vi "ABB global.vi"() -> ()   [LabVIEW 2017]
panel:
  in  "Temp report folder":path=path "C:/Program Files/National Instruments/LabVIEW 7.1/LabView 7.1 Apps/ABB motor test/report templates"
  in  "Camera Addresses":T1
  out "Video Display Folder":path
  in  "ChangeVIdStreamPath":path=path "C:/Program Files/National Instruments/LabVIEW 7.1/LabView 7.1 Apps/ABB motor test/report templates"
  in  "Temperature sensors":string[](array[string])
  in  "Efficiency Units":u16(ring) items=["METRIC", "IMPERIAL", "", "", ""]
  in  "Running Average levels (dB)":cluster{"Total":dbl, "Log":dbl}
  in  "Background Average levels (dB)":cluster{"Total":dbl, "Log":dbl}
  in  "Running Noise analysis":dbl[][](array[numeric])
  in  "Background Noise analysis":dbl[][](array[numeric])
  in  "Efficiency Standard":u16(ring) items=["IEC", "NEMA"]
  in  "Additional Mech Loss":dbl
  in  "Slip ring temperatures":cluster{"K":dbl, "L":dbl, "M ":dbl}[](array[cluster])
  in  "Specified Noise":dbl
  in  "Nose Limit":dbl
  in  "Effy Load Selection":bool[](array[boolean])
  in  "PF Remarks":string
  in  "Noise mtr type":i32
  in  "# noise points":i32
  in  "Heat run VT&CT":T2={"VT Primary"=0.0, "VT Secondary"=0.0, "CT  Primary"=0.0, "CT Secondary"=0.0, "Current Shunt"=enum."Internal", "Avg interval"=0.3}
  in  "Locked rotor VT&CT":T2={"VT Primary"=0.0, "VT Secondary"=0.0, "CT  Primary"=0.0, "CT Secondary"=0.0, "Current Shunt"=enum."Internal", "Avg interval"=0.3}
  in  "Noload VT&CT":T2={"VT Primary"=0.0, "VT Secondary"=0.0, "CT  Primary"=0.0, "CT Secondary"=0.0, "Current Shunt"=enum."Internal", "Avg interval"=0.3}
  in  "Webdaq Report":cluster{"Report":string, "Interval":string}={"Report"="Test_1", "Interval"="LastScan"}
  in  "Cool curve rdgs":T3(array[cluster])
  in  "report IDs":cluster{"Document #":string, "Revision":string}={"Document #"="1234H2345", "Revision"="1.1"}
  in  "VT and CT Ratios":T4={"VT Primary"=0.0, "VT Secondary"=0.0, "CT  Primary"=0.0, "CT Secondary"=0.0, "Current Shunt"=enum."Internal", "Averaging interval"=0.3}
  in  "Rotor Insulation Resistance":T5
  in  "Stator Insulation Resistance":T5
  in  "Heat run Type":enum16{"Full Load", "Partial- & No-Load"}(ring)
  in  "Altitude":dbl=1550.0
  in  "Max Wdg temp rise":dbl=85.0
  in  "No load run config":T6
  in  "Noise Levels":cluster{"Noise Before":dbl, "Noise During":dbl}
  in  "Pass Fail Entries":string[][](array[string])
  in  "Effiy entries":string[][](array[string])
  in  "Effy Configuration":T7 {"Loads (%Rated)" format="%#.0f"}
  in  "Temperature Scaling":dbl[][](array[numeric])
  in  "Bearing run config":T6
  in  "Instruments":string[][](array[string])
  in  "Heat run config":T6
  in  "Heat Run Results":cluster{"results":dbl[][], "Comments":string}[](array[cluster])
  in  "Personel":string[](array[string])
  in  "Tested by":string[](array[string])
  in  "Bearing Insp results":string[](array[string])
  in  "Bearing Image files":string[][](array[string])
  in  "Noise Image files":string[][](array[string])
  in  "Viewing test":bool
  in  "Current test":path
  in  "Report template":string
  in  "Noise results":dbl[][](array[numeric])
  in  "Bearing run results":dbl[][](array[numeric])
  in  "report template folder":path=path "C:/Program Files/National Instruments/LabVIEW 7.1/LabView 7.1 Apps/ABB motor test/report templates"
  in  "miscellaneous":string[](array[string])
  in  "Bearing Run Autordg":T8={"Thermal Stability (%)"=2.0, "Reading interval (mins)"=2.0}
  in  "Locked rotor temp. alloc":i32[](array[numeric])
  in  "NoLoad temp. alloc":i32[](array[numeric])
  in  "Temperature names":string[](array[string])
  in  "Temperature alloc":string[](array[string])
  in  "Heat Run Autordg":T9={"Thermal Stability (deg/hr)"=2.0, "Reading interval (mins)"=2.0}
  in  "Locked rotor test results":dbl[][](array[numeric])
  in  "Locked Rotor Autordg":T10={"Number Values"=8, "Tolerance"=2.0, "Value (ratio) "=[1.15, 1.0, 0.91, 0.78, 0.66, 0.55, 0.42, 0.3], "Hold time (sec)"=2.0}
  in  "No Load Autordg":T11={"Number Values"=8, "Tolerance "=2.0, "Value (ratio)"=[1.15, 1.0, 0.91, 0.78, 0.66, 0.55, 0.42, 0.3], "Hold time (sec)"=2.0}
  in  "Comments":string
  in  "No load test results":dbl[][](array[numeric])
  in  "Entered Data":string[][](table)
  in  "Results folder":path
  in  "System":T12={"Simulate Norma"=FALSE, "Norma 5000 Address"=5, "WebDaq IP Address"="", "Simulate cDAQ"=FALSE} {"Norma 5000 Address" min=1 max=31}
  in  "Start timeout":i32=30
  in  "Password":string
  # "with"
  # "at"
  # "with"
  # "at"
  # "with"
  # "at"
  # "with"
  # "at"
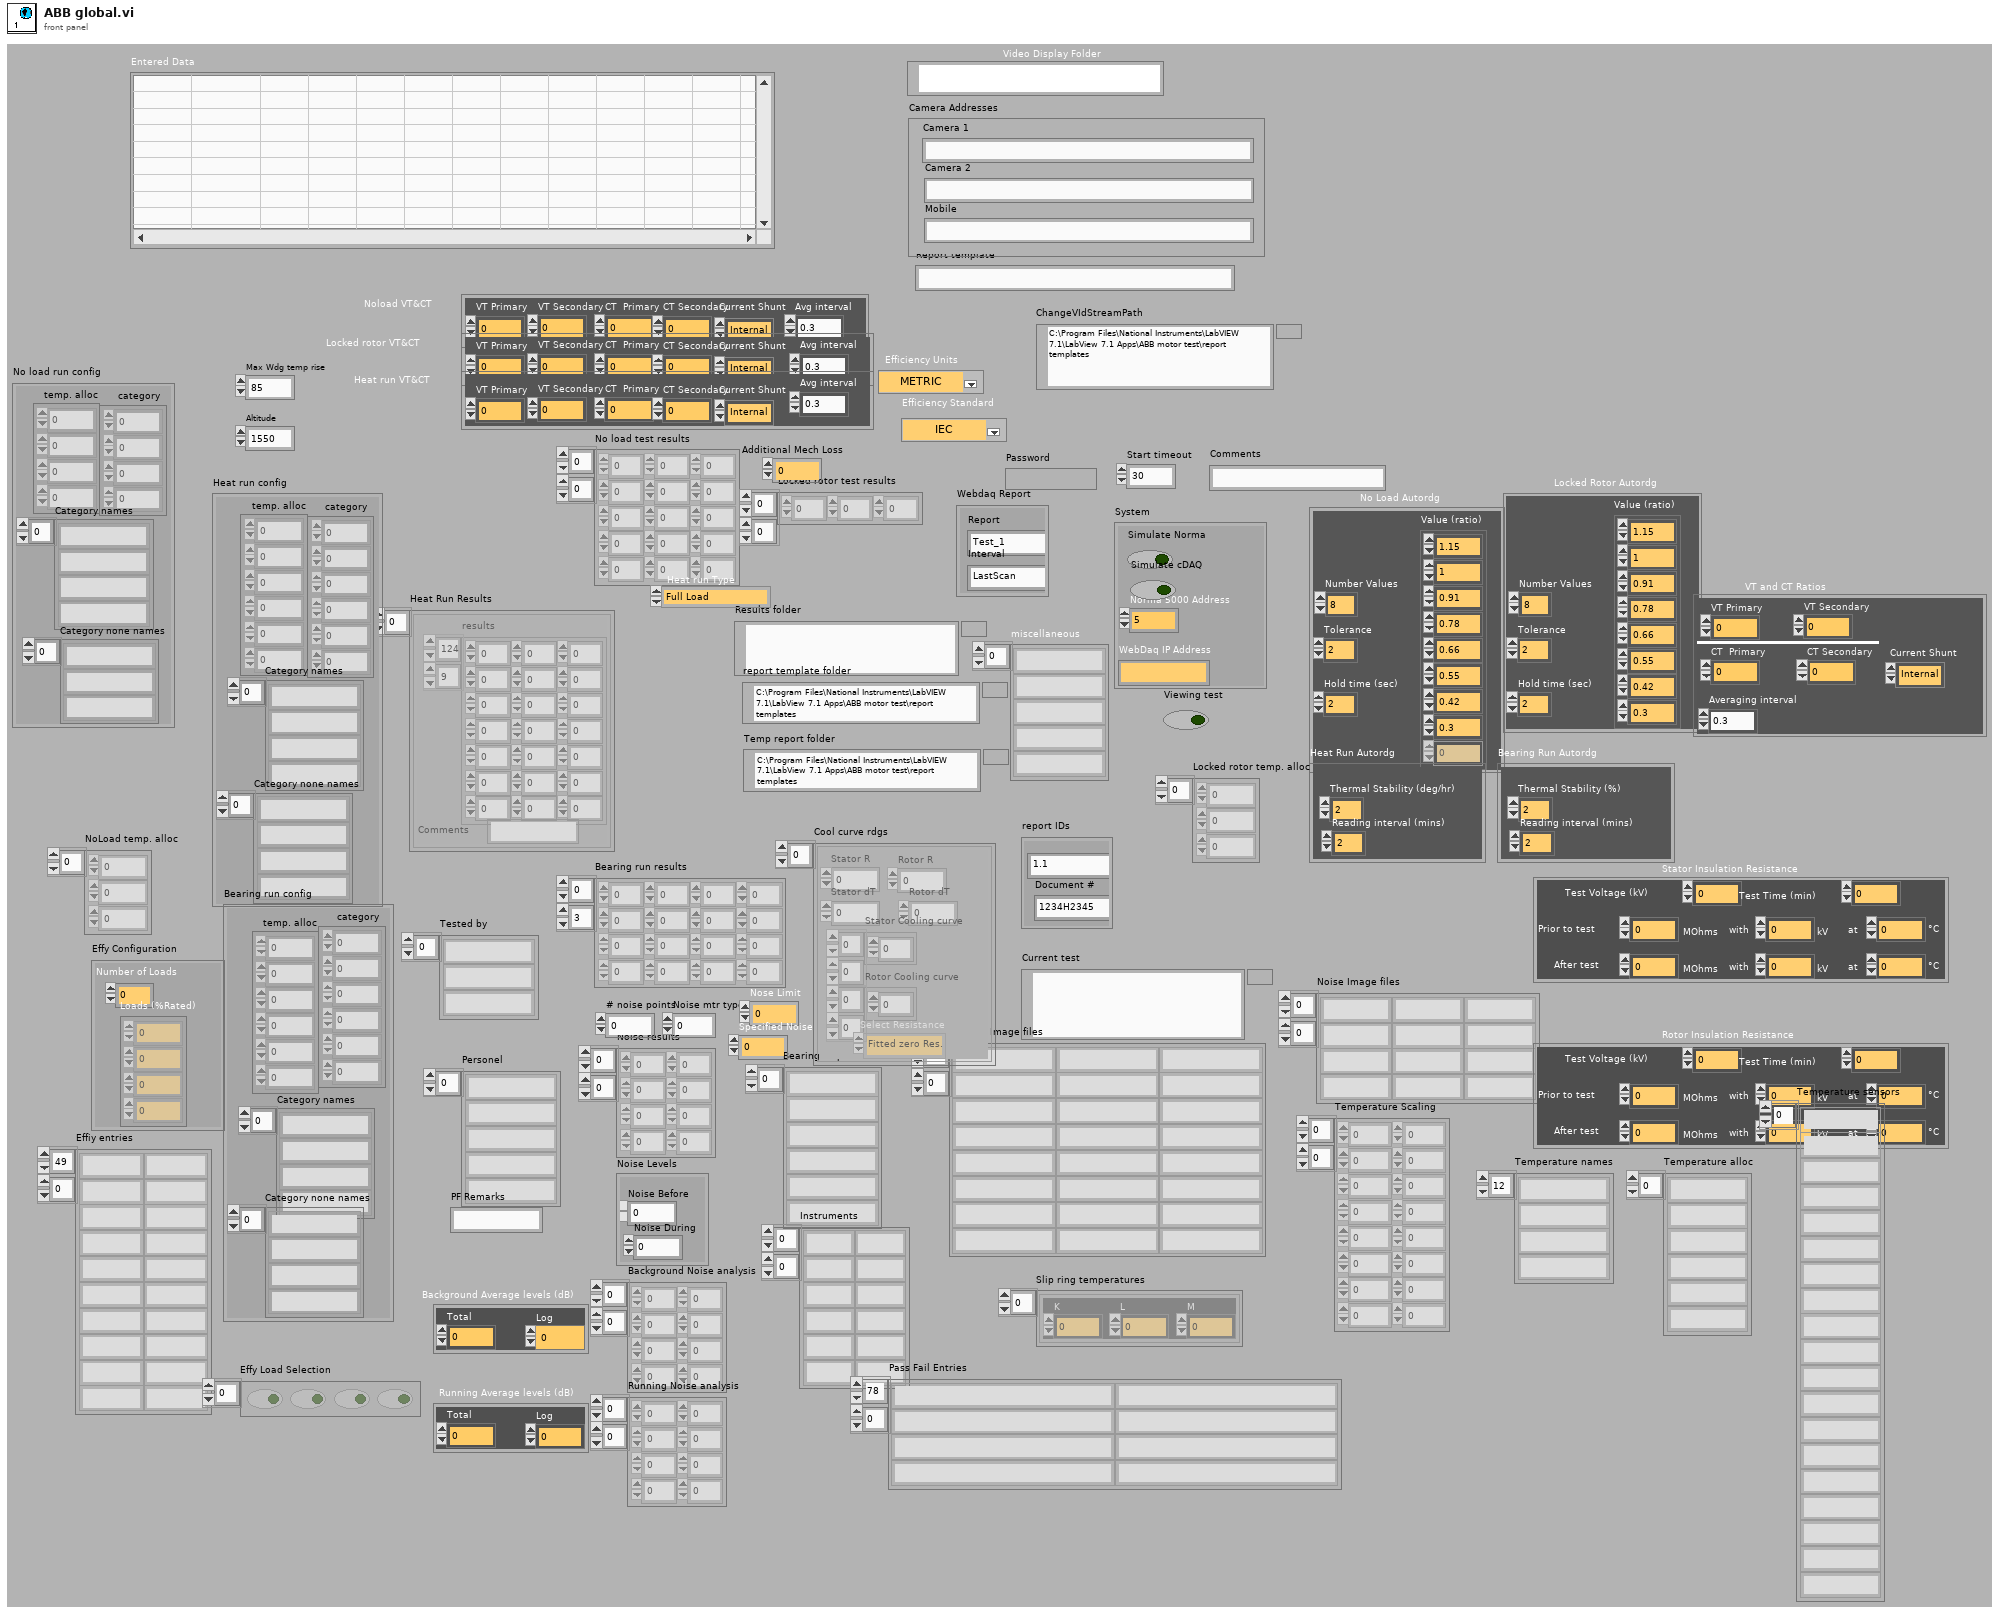
[diagram p1: front panel]
types:
  T1 = cluster{"Camera 1":string, "Camera 2":string, "Mobile":string}
  T2 = cluster{"VT Primary":dbl, "VT Secondary":dbl, "CT  Primary":dbl, "CT Secondary":dbl, "Current Shunt":enum16{"Internal", "External"}, "Avg interval":dbl}
  T3 = cluster{"Stator R":dbl, "Stator dT":dbl, "Rotor R":dbl, "Rotor dT":dbl, "Stator Cooling curve":dbl[][], "Rotor Cooling curve":dbl[][], "Select Resistance":enum16{"Fitted zero Res.", "Selected Res.", "Entered Res."}}[]
  T4 = cluster{"VT Primary":dbl, "VT Secondary":dbl, "CT  Primary":dbl, "CT Secondary":dbl, "Current Shunt":enum16{"Internal", "External"}, "Averaging interval":dbl}
  T5 = cluster{"Prior to test":dbl, "Prior v":dbl, "Prior temp":dbl, "After test":dbl, "after v":dbl, "After temp":dbl, "Test Voltage (kV)":dbl, "Test Time (min)":dbl}
  T6 = cluster{"temp. alloc":i32[], "category":i32[], "Category names":string[], "Category none names":string[]}
  T7 = cluster{"Number of Loads":i32, "Loads (%Rated)":dbl[]}
  T8 = cluster{"Thermal Stability (%)":dbl, "Reading interval (mins)":dbl}
  T9 = cluster{"Thermal Stability (deg/hr)":dbl, "Reading interval (mins)":dbl}
  T10 = cluster{"Number Values":i32, "Tolerance":dbl, "Value (ratio) ":dbl[], "Hold time (sec)":dbl}
  T11 = cluster{"Number Values":i32, "Tolerance ":dbl, "Value (ratio)":dbl[], "Hold time (sec)":dbl}
  T12 = cluster{"Simulate Norma":bool, "Norma 5000 Address":u8, "WebDaq IP Address":string, "Simulate cDAQ":bool}
diagram:
